vi "Move Elves.vi"(10 "propose Moves":T2, 11 "Elf Positions":T1[](array[typedef])) -> (3 "New Elf Positions":T1[](array[typedef]))   [LabVIEW 2023]
uses:
  MAP_Poroposed Moves.ctl
  Cluster _Point Location.ctl
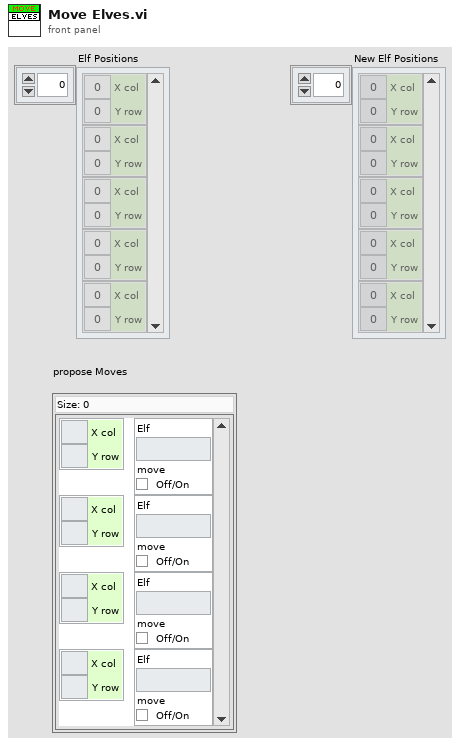
[diagram p1: front panel]
types:
  T1 = typedef "Cluster _Point Location.ctl" = cluster{"X col":i32, "Y row":i32}
  T2 = typedef "MAP_Poroposed Moves.ctl" = map{T1, cluster{"Elf":i32, "move":bool}}
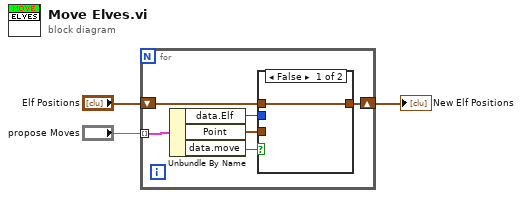
[diagram p0: block diagram]
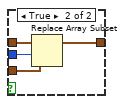
[diagram p2: hidden frame]
diagram:
  n1 = for {
    tunnel: "propose Moves" -> [w9] mode=indexing
    shift-right: [w5] -> w1
    shift-left: "Elf Positions" -> [w7]
    n2 = Unbundle By Name(w9) -> ("data.Elf"=w4:i32, "Point"=w6:T1, "data.move"=w8:bool)
    n3 = case shown="False" w8 {
      tunnel: w7 -> [w10 w14]
      tunnel: w6 -> [_ w11]
      tunnel: [w10 w13] -> w5
      tunnel: w4 -> [_ w12]
      frame False {
      }
      frame True {
        n4 = Replace Array Subset(array=w14, new element=w11, index=w12) -> (w13:T1[])
      }
    }
  }
  "New Elf Positions" <- w1
